vi "Pre Build Icon Editor PPL.vi"(6 "Top Level/Always Included VIs":path[](array[path]), 7 "Main Destination Path":path, 9 "Target Name":string, 10 "Build Specification Name":string, 11 "Project Path":path) -> (0 "error out":errorcluster)   [LabVIEW 2020]
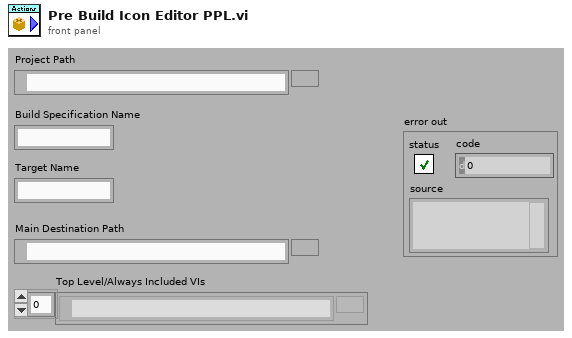
[diagram p1: front panel]
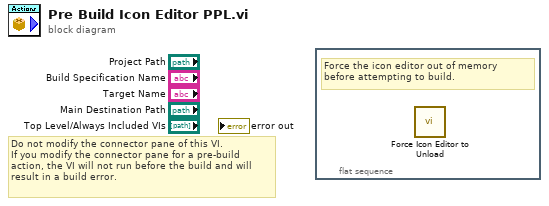
[diagram p0: block diagram]
diagram:
  # "Do not modify the connector pane of this VI. \nIf you modify the connector pane for a pre-build\naction, the VI will not run before the build and will\nresult in a build error."
  n1 = flat-sequence {
    frame #0 {
      # "Force the icon editor out of memory\nbefore attempting to build."
      n2 = call "Force Icon Editor to Unload.vi"() -> ()  [unwired: 12 in]
    }
  }
